vi "Trans_FPGA-old.vi"() -> ()   [LabVIEW 2016]
uses:
  <vilib>/eio/EIONode/EIONode.xnode
  <vilib>/eio/EIOMethodNode/EIOMethodNode.xnode
  <vilib>/LabVIEW Targets/FPGA/cRIO/shared/nicrio_ModuleControls/nicrio_cRIO-9871_BaudRateEnum.ctl
  <vilib>/LabVIEW Targets/FPGA/cRIO/shared/nicrio_ModuleControls/nicrio_cRIO-9871_DataBitsEnum.ctl
  <vilib>/LabVIEW Targets/FPGA/cRIO/shared/nicrio_ModuleControls/nicrio_cRIO-9871_ParityEnum.ctl
  <vilib>/LabVIEW Targets/FPGA/cRIO/shared/nicrio_ModuleControls/nicrio_cRIO-9871_StopBitsEnum.ctl
  <vilib>/eio/EIOPropertyNode/EIOPropertyNode.xnode
  <vilib>/rvi/Analysis/measure/dc-rms/XNode/niFpgaDC-RMS.xnode
  <vilib>/rvi/eio/common/nirviEmuTemplateMethod_errors.vi
  <vilib>/Platform/TimedLoop/XDataNode/wakeup.ctl
  <vilib>/Platform/TimedLoop/XDataNode/XDNodeRunTimeDep.lvlib
  <vilib>/Platform/TimedLoop/XDataNode/nitl_modes.ctl
  <vilib>/Platform/TimedLoop/XDataNode/timing_clust.ctl
  <vilib>/Platform/TimedLoop/XDataNode/XDataNode.xnode
  <vilib>/rvi/FXPMathLib/basic elements/FxpIntAccumulator/XNode/nifxpmath_IntAccumulator.xnode
  <vilib>/rvi/FXPMathLib/FxpMul/XNode/nifxpmath_Multiplier.xnode
  <vilib>/rvi/Analysis/common/codeGenErrors/XNode/niFpgaXNodeCodeGenErrorHandle.vi
  <vilib>/rvi/FXPMathLib/basic elements/FxpIntAccumulator/simVIs/DllFxpIntAccumulator_sub.vi
  <vilib>/rvi/FXPMathLib/basic elements/FxpIntAccumulator/subVIs/nifxpmath_IntAccumulator_SimConfig.ctl
  <vilib>/rvi/FXPMathLib/sim/FxpSim.dll
  <vilib>/rvi/eio/common/nirviEmuTemplatePropertyGet_errors.vi
  <vilib>/rvi/eio/common/nirviEmuTemplatePropertyGet_noerrors.vi
  <vilib>/rvi/eio/common/nirviEmuTemplatePropertySet_errors.vi
  <vilib>/rvi/eio/common/nirviEmuTemplatePropertySet_noerrors.vi
panel:
  in  "analyze ps set array":u8[](array[numeric])=[0, 0, 0, 0, 0, 0, 0, 0, 0, 0]
  out "Data":u8
  out "Timed Out":bool
  out "Analyze read":u8[](array[numeric])
  out "error out":errorcluster
  out "Ion gauge 4":u8[](array[numeric])
  out "Convectron 4":u8[](array[numeric])
  out "Convectron 3":u8[](array[numeric])
  out "Ion gauge 3":u8[](array[numeric])
  out "Ion gauge 2":u8[](array[numeric])
  out "Convectron 2":u8[](array[numeric])
  out "Convectron 1":u8[](array[numeric])
  out "Ion gauge 1":u8[](array[numeric])
  in  "Analog Output":fxp<+/-,26,5>[](array[numeric])=[0.0, 0.0, 0.0, 0.0, 0.0, 0.0, 0.0, 0.0] format="%.23g"
  out "Analog input":fxp<+/-,26,5>[](array[numeric]) format="%.23g"
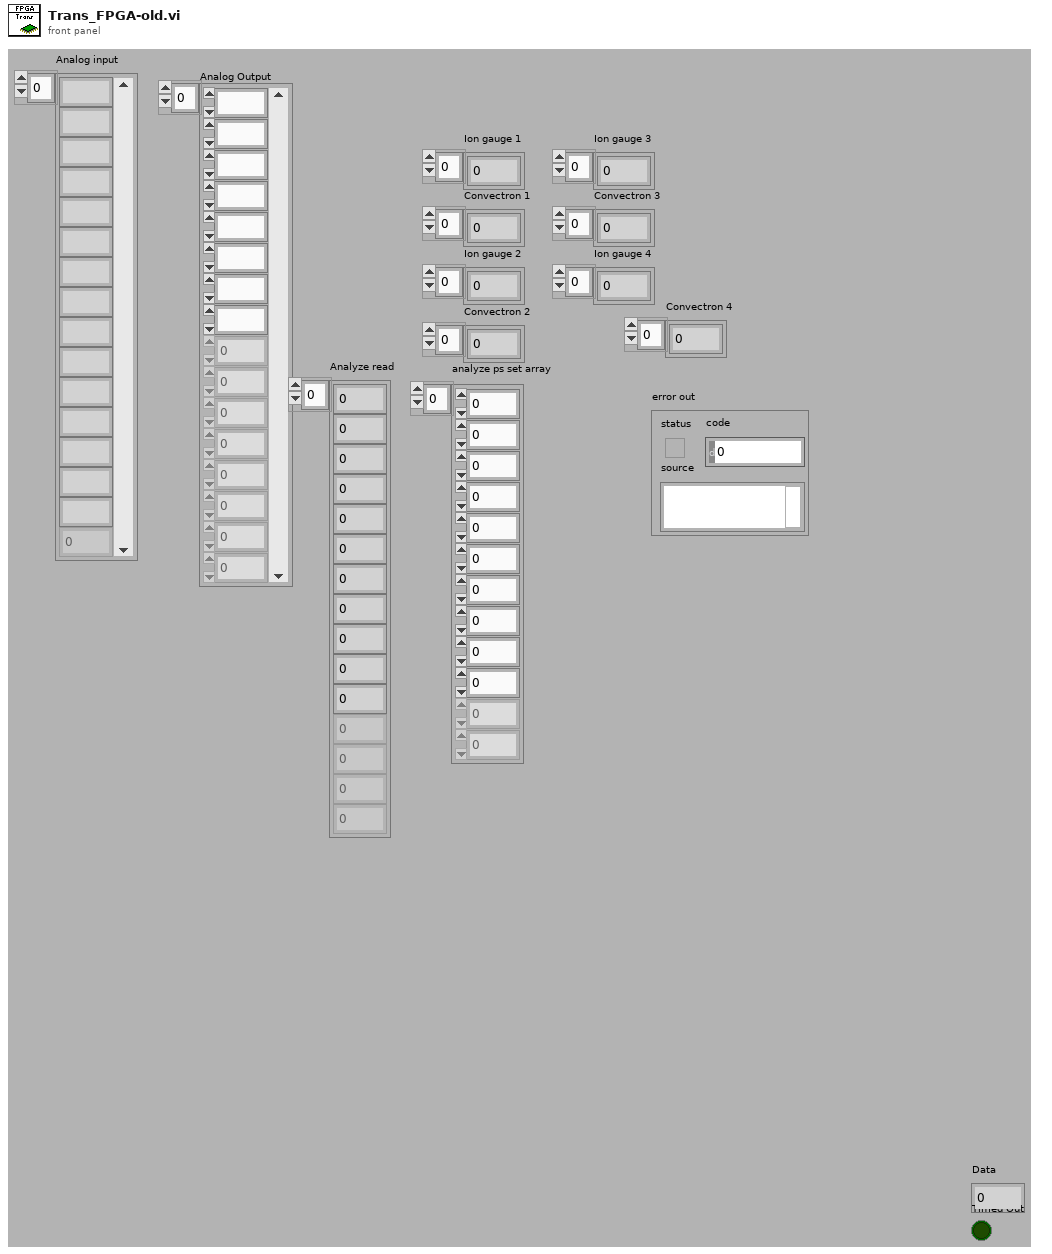
[diagram p1: front panel]
types:
  T1 = typedef "nicrio_cRIO-9871_StopBitsEnum.ctl" = enum8{"1", "1.5", "2"}
  T2 = typedef "nicrio_cRIO-9871_BaudRateEnum.ctl" = enum16{"75 bps", "110 bps", "134 bps", "150 bps", "300 bps", "600 bps", "1200 bps", "1800 bps", "2400 bps", "4800 bps", "7200 bps", "9600 bps", "14.4 kbps", "19.2 kbps", "28.8 kbps", "38.4 kbps", "57.6 kbps", "115.2 kbps", "230.4 kbps", "460.8 kbps", "921.6 kbps"}
  T3 = typedef "nicrio_cRIO-9871_ParityEnum.ctl" = enum8{"None", "Odd", "Even", "Mark", "Space"}
  T4 = typedef "nicrio_cRIO-9871_DataBitsEnum.ctl" = enum8{"5", "6", "7", "8"}
  T5 = typedef "XDNodeRunTimeDep.lvlib/timing_clust.ctl" = cluster{"Expected End [f-1]":u64, "Actual End [f-1]":u64, "Finished Late? [f-1]":bool, "Expected End [i-1]":u64, "Actual End [i-1]":u64, "Finished Late? [i-1]":bool, "Expected Start [i]":u64, "Actual Start [i]":u64, "Expected Start [f]":u64, "Actual Start [f]":u64, "Source Name":string, "Structure Name":string, "Period":i64, "Deadline":i64, "Offset":i64, "Start":i64, "Priority":i32, "Timeout":i32, "Mode":T6, "Wakeup Reason":T7, "Error":errorcluster, "Source Type":string, "Secondary Source Type":string, "Global End Time":u64, "Global Start Time":u64, "Frame Duration":u64, "Iteration Duration":u64, "Assigned CPU":i32, "I/O Scan Engine Mode":u32}
  T6 = typedef "XDNodeRunTimeDep.lvlib/nitl_modes.ctl" = enum32{"No Change", "Process missed periods, maintain original phase", "Discard missed periods, maintain original phase", "Process missed periods, ignore original phase", "Discard missed periods, ignore original phase"}
  T7 = typedef "XDNodeRunTimeDep.lvlib/wakeup.ctl" = enum32{"Normal", "Aborted", "Asynchronous wakeup", "Timing source error", "Timed loop error", "Timeout"}
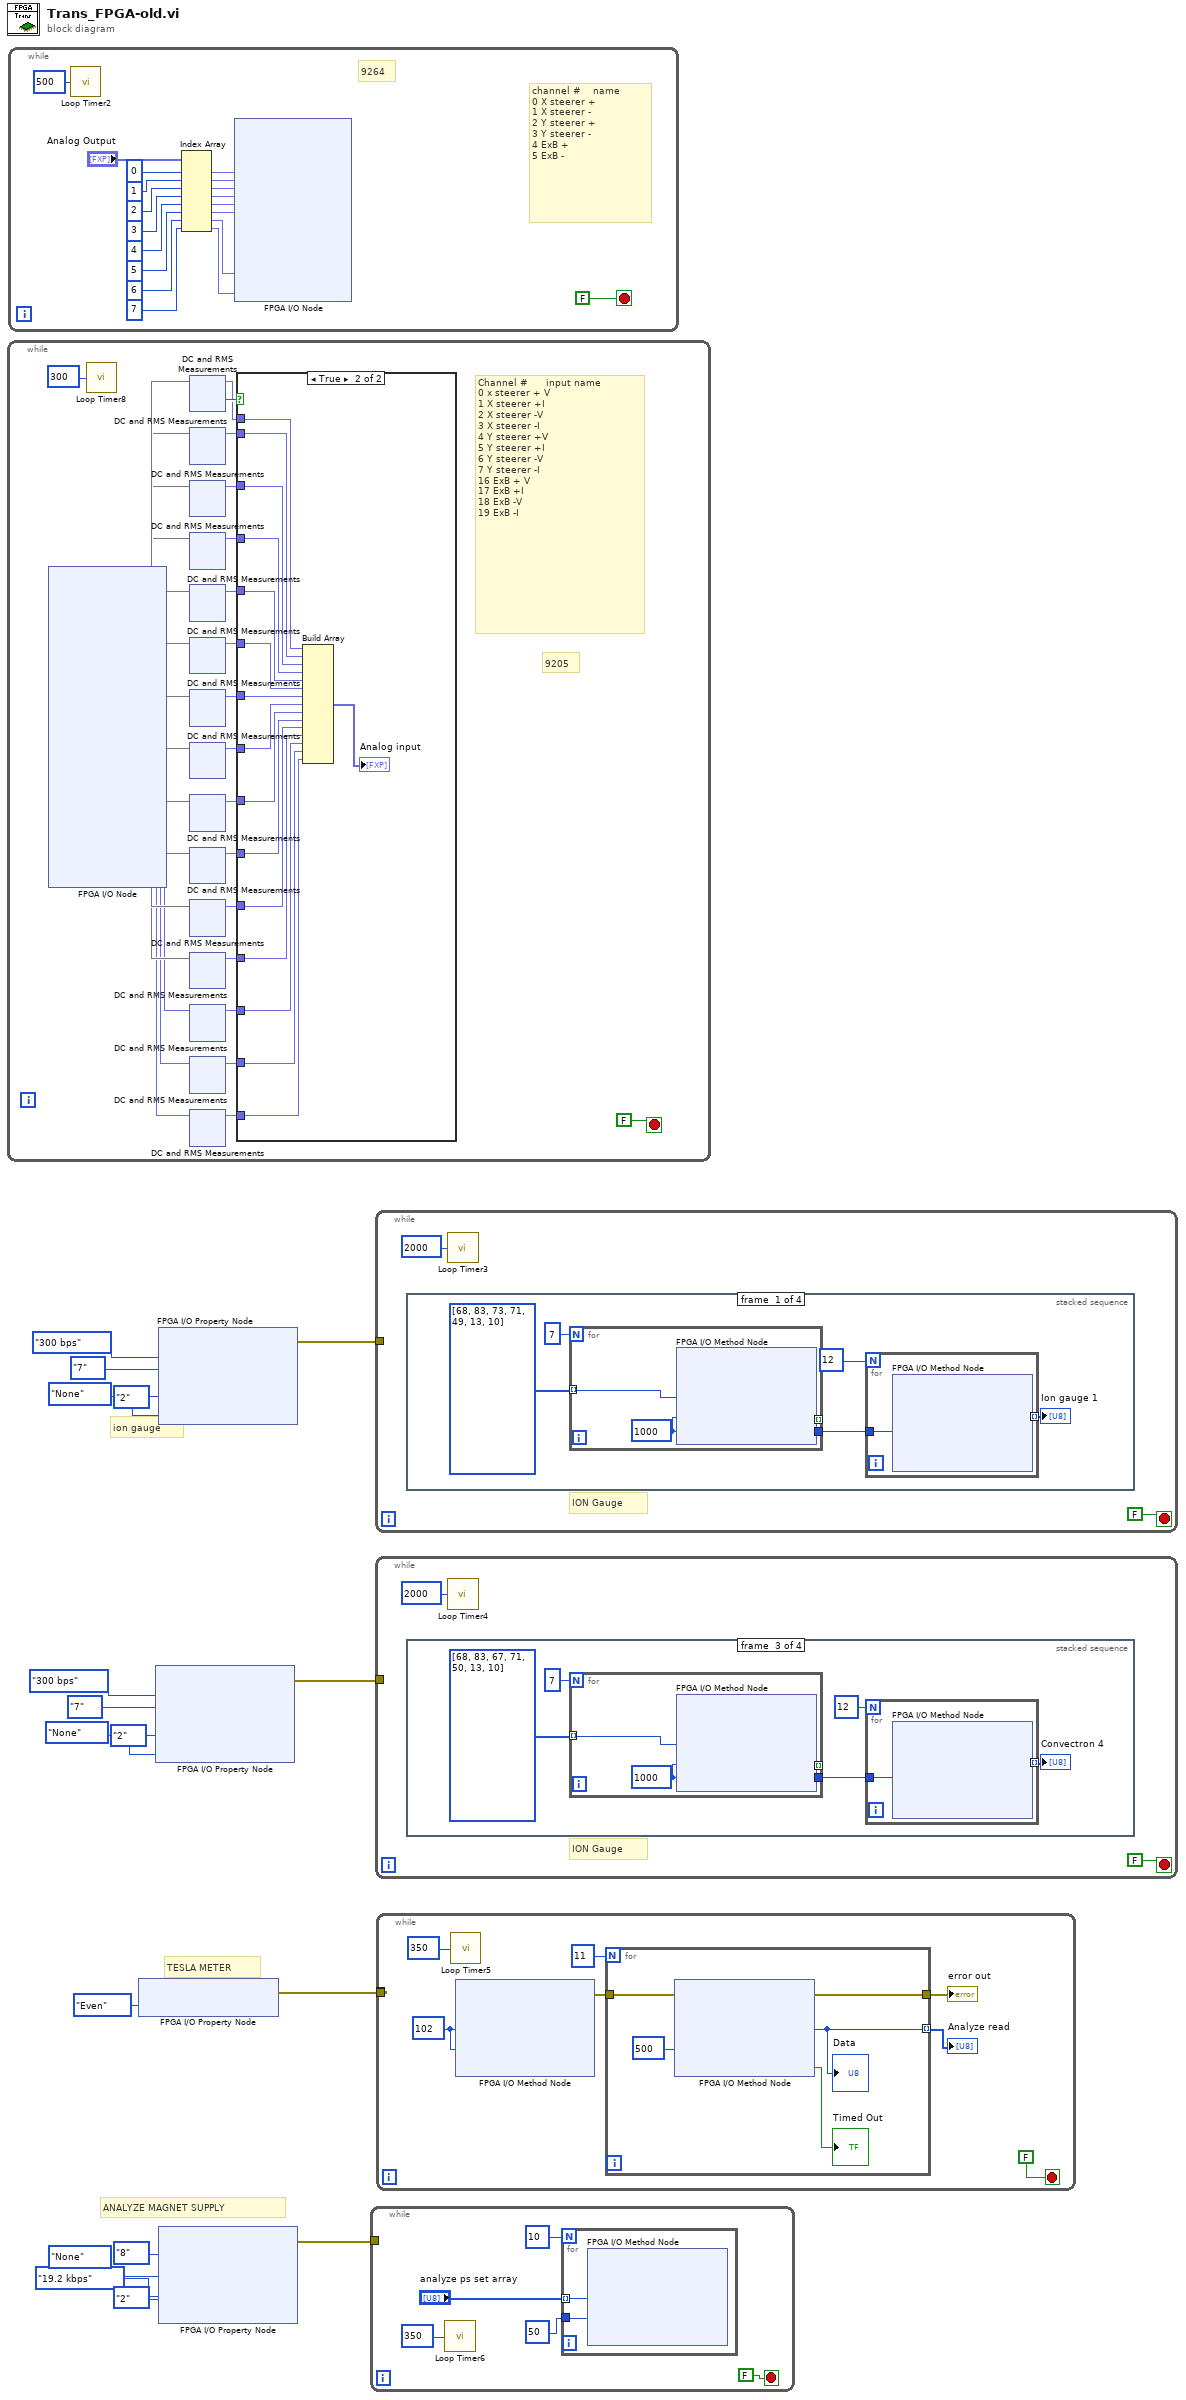
[diagram p0: block diagram]
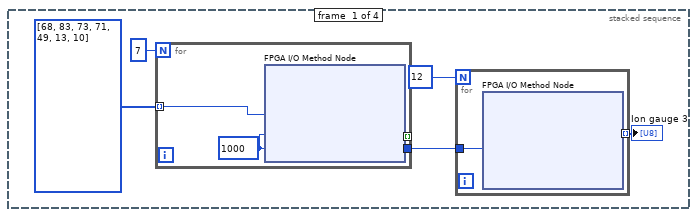
[diagram p3: hidden frame]
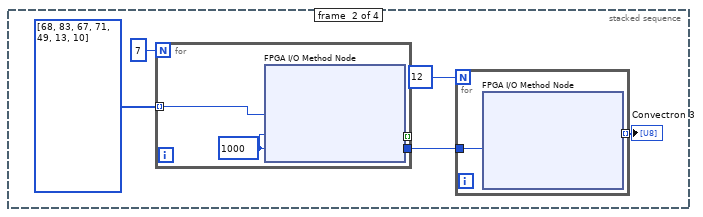
[diagram p4: hidden frame]
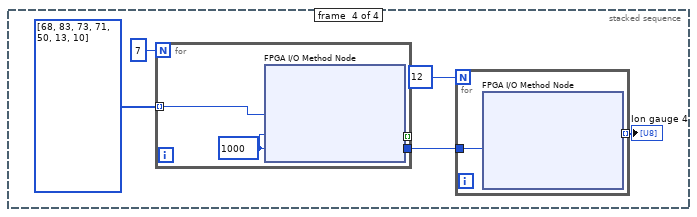
[diagram p5: hidden frame]
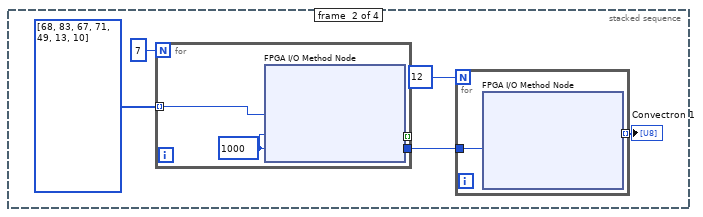
[diagram p6: hidden frame]
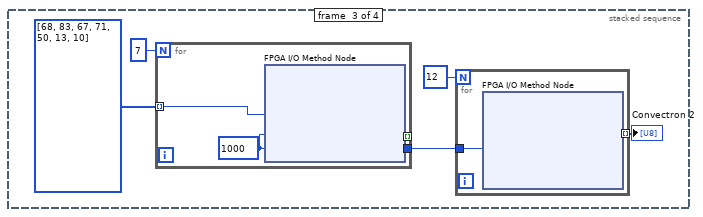
[diagram p7: hidden frame]
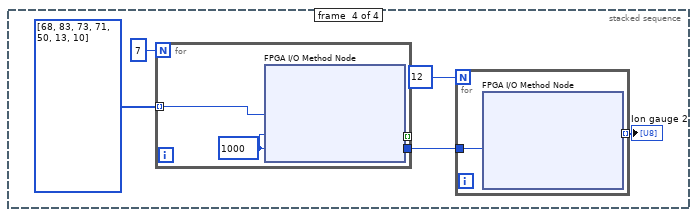
[diagram p8: hidden frame]
diagram:
  # "ANALYZE MAGNET SUPPLY"
  # "TESLA METER"
  # "ion gauge"
  n1 = while {
    stop <- FALSE stop-if-true
    # "Channel #      input name\n0 x steerer + V\n1 X steerer +I\n2 X steerer -V\n3 X steerer -I\n4 Y steerer +V\n5 Y steerer +I\n6 Y steerer -V\n7 Y steerer -I\n16 ExB + V\n17 ExB +I\n18 ExB -V\n19 ExB -I"
    # "9205"
    n2 = xnode "FPGA I/O Node"() -> ("Mod2/AI0"=w47, "Mod2/AI1"=w45, "Mod2/AI2"=w43, "Mod2/AI3"=w41, "Mod2/AI4"=w39, "Mod2/AI5"=w37, "Mod2/AI6"=w35, "Mod2/AI7"=w33, "Mod2/AI16"=w31, "Mod2/AI17"=w29, "Mod2/AI18"=w27, "Mod2/AI19"=w25, "Mod2/AI20"=w23:fxp<+/-,26,5>, "Mod2/AI21"=w21:fxp<+/-,26,5>, "Mod2/AI22"=w19:fxp<+/-,26,5>)  [unwired: 15 in, 15 out]
    n3 = call "Loop Timer8"("Count(Ticks)"=u32 300) -> ()  [unwired: 1 out]
    n4 = xnode "DC and RMS Measurements"("input data"=w47) -> ("DC"=w46:fxp<+/-,26,5>, "output valid"=w48:bool)  [unwired: 1 in]
    n5 = xnode "DC and RMS Measurements"("input data"=w45) -> ("DC"=w44:fxp<+/-,26,5>)  [unwired: 1 in, 1 out]
    n6 = xnode "DC and RMS Measurements"("input data"=w43) -> ("DC"=w42:fxp<+/-,26,5>)  [unwired: 1 in, 1 out]
    n7 = xnode "DC and RMS Measurements"("input data"=w41) -> ("DC"=w40:fxp<+/-,26,5>)  [unwired: 1 in, 1 out]
    n8 = xnode "DC and RMS Measurements"("input data"=w39) -> ("DC"=w38:fxp<+/-,26,5>)  [unwired: 1 in, 1 out]
    n9 = xnode "DC and RMS Measurements"("input data"=w37) -> ("DC"=w36:fxp<+/-,26,5>)  [unwired: 1 in, 1 out]
    n10 = xnode "DC and RMS Measurements"("input data"=w35) -> ("DC"=w34:fxp<+/-,26,5>)  [unwired: 1 in, 1 out]
    n11 = xnode "DC and RMS Measurements"("input data"=w33) -> ("DC"=w32:fxp<+/-,26,5>)  [unwired: 1 in, 1 out]
    n12 = xnode "DC and RMS Measurements"("input data"=w31) -> ("DC"=w30:fxp<+/-,26,5>)  [unwired: 1 in, 1 out]
    n13 = xnode "DC and RMS Measurements"("input data"=w29) -> ("DC"=w28:fxp<+/-,26,5>)  [unwired: 1 in, 1 out]
    n14 = xnode "DC and RMS Measurements"("input data"=w27) -> ("DC"=w26:fxp<+/-,26,5>)  [unwired: 1 in, 1 out]
    n15 = xnode "DC and RMS Measurements"("input data"=w25) -> ("DC"=w24:fxp<+/-,26,5>)  [unwired: 1 in, 1 out]
    n16 = xnode "DC and RMS Measurements"("input data"=w23) -> ("DC"=w22:fxp<+/-,26,5>)  [unwired: 1 in, 1 out]
    n17 = xnode "DC and RMS Measurements"("input data"=w21) -> ("DC"=w20:fxp<+/-,26,5>)  [unwired: 1 in, 1 out]
    n18 = xnode "DC and RMS Measurements"("input data"=w19) -> ("DC"=w18:fxp<+/-,26,5>)  [unwired: 1 in, 1 out]
    n19 = case shown="True" w48 {
      tunnel: w46 -> [_ w226]
      tunnel: w44 -> [_ w225]
      tunnel: w42 -> [_ w224]
      tunnel: w40 -> [_ w223]
      tunnel: w38 -> [_ w222]
      tunnel: w36 -> [_ w221]
      tunnel: w34 -> [_ w220]
      tunnel: w32 -> [_ w219]
      tunnel: w30 -> [_ w218]
      tunnel: w28 -> [_ w217]
      tunnel: w26 -> [_ w216]
      tunnel: w24 -> [_ w215]
      tunnel: w22 -> [_ w214]
      tunnel: w20 -> [_ w213]
      tunnel: w18 -> [_ w212]
      frame False {
      }
      frame True {
        n20 = Build Array(w226, w225, w224, w223, w222, w221, w220, w219, w218, w217, w216, w215, w214, w213, w212) -> (→"Analog input":fxp<+/-,26,5>[])
      }
    }
  }
  n21 = while {
    stop <- FALSE stop-if-true
    # "channel #    name\n0 X steerer +\n1 X steerer -\n2 Y steerer +\n3 Y steerer -\n4 ExB +\n5 ExB -"
    # "9264"
    n22 = call "Loop Timer2"("Count(uSec)"=u32 500 ("Count(Ticks)")) -> ()  [unwired: 1 out]
    n23 = Index Array(array="Analog Output", index #1=0 ("index"), index #2=1 ("index"), index #3=2 ("index"), index #4=3 ("index"), index #5=4 ("index"), index #6=5 ("index"), index #7=6 ("index"), index #8=7 ("index")) -> (element #1=w1278:fxp<+/-,26,5>, element #2=w1277:fxp<+/-,26,5>, element #3=w1276:fxp<+/-,26,5>, element #4=w1275:fxp<+/-,26,5>, element #5=w1270:fxp<+/-,26,5>, element #6=w1269:fxp<+/-,26,5>, element #7=w1268:fxp<+/-,26,5>, element #8=w1267:fxp<+/-,26,5>)
    n24 = xnode "FPGA I/O Node"("Mod1/AO0"=w1278, "Mod1/AO1"=w1277, "Mod1/AO2"=w1276, "Mod1/AO3"=w1275, "Mod1/AO4"=w1270, "Mod1/AO5"=w1269, "Mod1/AO6"=w1268, "Mod1/AO7"=w1267) -> ()  [unwired: 8 in, 8 out]
  }
  n25 = xnode "FPGA I/O Property Node"("Parity"=nicrio_cRIO-9871_ParityEnum."Even") -> ("error out"=w2:errorcluster)  [unwired: 2 in, 1 out]
  n26 = xnode "FPGA I/O Property Node"("Baud Rate"=nicrio_cRIO-9871_BaudRateEnum."300 bps", "Data Bits"=nicrio_cRIO-9871_DataBitsEnum."7", "Parity"=nicrio_cRIO-9871_ParityEnum."None", "Stop Bits"=nicrio_cRIO-9871_StopBitsEnum."2") -> ("error out"=w3:errorcluster)  [unwired: 2 in, 1 out]
  n27 = xnode "FPGA I/O Property Node"("Baud Rate"=nicrio_cRIO-9871_BaudRateEnum."300 bps", "Data Bits"=nicrio_cRIO-9871_DataBitsEnum."7", "Parity"=nicrio_cRIO-9871_ParityEnum."None", "Stop Bits"=nicrio_cRIO-9871_StopBitsEnum."2") -> ("error out"=w4:errorcluster)  [unwired: 2 in, 1 out]
  n28 = xnode "FPGA I/O Property Node"("Data Bits"=nicrio_cRIO-9871_DataBitsEnum."8", "Parity"=nicrio_cRIO-9871_ParityEnum."None", "Baud Rate"=nicrio_cRIO-9871_BaudRateEnum."19.2 kbps", "Stop Bits"=nicrio_cRIO-9871_StopBitsEnum."2") -> ("error out"=w1:errorcluster)  [unwired: 2 in, 1 out]
  n29 = while {
    tunnel: w1 -> [_]
    stop <- FALSE stop-if-true
    n30 = call "Loop Timer6"("Count(mSec)"=u32 350) -> ()  [unwired: 1 out]
    n31 = for {
      N: 10 -> [_]
      tunnel: 50 ("Timeout (ms)") -> [w1292]
      tunnel: "analyze ps set array" -> [w1291] mode=indexing
      n32 = xnode "FPGA I/O Method Node"("Data"=w1291, "Timeout (ms)"=w1292) -> ()  [unwired: 2 in, 3 out]
    }
  }
  n33 = while {
    tunnel: w4 -> [_]
    stop <- FALSE stop-if-true
    # "ION Gauge"
    n34 = stacked-sequence {
      frame #0 {
        n35 = for {
          N: 7 -> [_]
          tunnel: [w1304] -> w1299
          tunnel: [w1303] -> _ mode=indexing
          tunnel: u8[] [68, 83, 73, 71, 49, 13, 10] ("unsigned byte array") -> [w1302] mode=indexing
          w1304 = 1000 ("Timeout (ms)")
          n36 = xnode "FPGA I/O Method Node"("Data"=w1302, "Timeout (ms)"=w1304) -> ("Timed Out"=w1303:bool)  [unwired: 1 in, 1 out]
        }
        n37 = for {
          N: 12 -> [_]
          tunnel: w1299 -> [w1301]
          tunnel: [w1300] -> w1295 mode=indexing
          n38 = xnode "FPGA I/O Method Node"("Timeout (ms)"=w1301) -> ("Data"=w1300:u8)  [unwired: 1 in, 2 out]
        }
        "Ion gauge 1" <- w1295
      }
      frame #1 {
        n39 = for {
          N: 7 -> [_]
          tunnel: [w1314] -> w1309
          tunnel: [w1313] -> _ mode=indexing
          tunnel: u8[] [68, 83, 67, 71, 49, 13, 10] ("unsigned byte array") -> [w1312] mode=indexing
          w1314 = 1000 ("Timeout (ms)")
          n40 = xnode "FPGA I/O Method Node"("Data"=w1312, "Timeout (ms)"=w1314) -> ("Timed Out"=w1313:bool)  [unwired: 1 in, 1 out]
        }
        n41 = for {
          N: 12 -> [_]
          tunnel: w1309 -> [w1311]
          tunnel: [w1310] -> w1305 mode=indexing
          n42 = xnode "FPGA I/O Method Node"("Timeout (ms)"=w1311) -> ("Data"=w1310:u8)  [unwired: 1 in, 2 out]
        }
        "Convectron 1" <- w1305
      }
      frame #2 {
        n43 = for {
          N: 7 -> [_]
          tunnel: [w1324] -> w1319
          tunnel: [w1323] -> _ mode=indexing
          tunnel: u8[] [68, 83, 67, 71, 50, 13, 10] ("unsigned byte array") -> [w1322] mode=indexing
          w1324 = 1000 ("Timeout (ms)")
          n44 = xnode "FPGA I/O Method Node"("Data"=w1322, "Timeout (ms)"=w1324) -> ("Timed Out"=w1323:bool)  [unwired: 1 in, 1 out]
        }
        n45 = for {
          N: 12 -> [_]
          tunnel: w1319 -> [w1321]
          tunnel: [w1320] -> w1315 mode=indexing
          n46 = xnode "FPGA I/O Method Node"("Timeout (ms)"=w1321) -> ("Data"=w1320:u8)  [unwired: 1 in, 2 out]
        }
        "Convectron 2" <- w1315
      }
      frame #3 {
        n47 = for {
          N: 7 -> [_]
          tunnel: [w1334] -> w1329
          tunnel: [w1333] -> _ mode=indexing
          tunnel: u8[] [68, 83, 73, 71, 50, 13, 10] ("unsigned byte array") -> [w1332] mode=indexing
          w1334 = 1000 ("Timeout (ms)")
          n48 = xnode "FPGA I/O Method Node"("Data"=w1332, "Timeout (ms)"=w1334) -> ("Timed Out"=w1333:bool)  [unwired: 1 in, 1 out]
        }
        n49 = for {
          N: 12 -> [_]
          tunnel: w1329 -> [w1331]
          tunnel: [w1330] -> w1325 mode=indexing
          n50 = xnode "FPGA I/O Method Node"("Timeout (ms)"=w1331) -> ("Data"=w1330:u8)  [unwired: 1 in, 2 out]
        }
        "Ion gauge 2" <- w1325
      }
    }
    n51 = call "Loop Timer3"("Count(mSec)"=u32 2000 ("Count(Ticks)")) -> ()  [unwired: 1 out]
  }
  n52 = while {
    tunnel: w3 -> [_]
    stop <- FALSE stop-if-true
    # "ION Gauge"
    n53 = stacked-sequence {
      frame #0 {
        n54 = for {
          N: 7 -> [_]
          tunnel: [w1346] -> w1341
          tunnel: [w1345] -> _ mode=indexing
          tunnel: u8[] [68, 83, 73, 71, 49, 13, 10] ("unsigned byte array") -> [w1344] mode=indexing
          w1346 = 1000 ("Timeout (ms)")
          n55 = xnode "FPGA I/O Method Node"("Data"=w1344, "Timeout (ms)"=w1346) -> ("Timed Out"=w1345:bool)  [unwired: 1 in, 1 out]
        }
        n56 = for {
          N: 12 -> [_]
          tunnel: w1341 -> [w1343]
          tunnel: [w1342] -> w1337 mode=indexing
          n57 = xnode "FPGA I/O Method Node"("Timeout (ms)"=w1343) -> ("Data"=w1342:u8)  [unwired: 1 in, 2 out]
        }
        "Ion gauge 3" <- w1337
      }
      frame #1 {
        n58 = for {
          N: 7 -> [_]
          tunnel: [w1356] -> w1351
          tunnel: [w1355] -> _ mode=indexing
          tunnel: u8[] [68, 83, 67, 71, 49, 13, 10] ("unsigned byte array") -> [w1354] mode=indexing
          w1356 = 1000 ("Timeout (ms)")
          n59 = xnode "FPGA I/O Method Node"("Data"=w1354, "Timeout (ms)"=w1356) -> ("Timed Out"=w1355:bool)  [unwired: 1 in, 1 out]
        }
        n60 = for {
          N: 12 -> [_]
          tunnel: w1351 -> [w1353]
          tunnel: [w1352] -> w1347 mode=indexing
          n61 = xnode "FPGA I/O Method Node"("Timeout (ms)"=w1353) -> ("Data"=w1352:u8)  [unwired: 1 in, 2 out]
        }
        "Convectron 3" <- w1347
      }
      frame #2 {
        n62 = for {
          N: 7 -> [_]
          tunnel: [w1366] -> w1361
          tunnel: [w1365] -> _ mode=indexing
          tunnel: u8[] [68, 83, 67, 71, 50, 13, 10] ("unsigned byte array") -> [w1364] mode=indexing
          w1366 = 1000 ("Timeout (ms)")
          n63 = xnode "FPGA I/O Method Node"("Data"=w1364, "Timeout (ms)"=w1366) -> ("Timed Out"=w1365:bool)  [unwired: 1 in, 1 out]
        }
        n64 = for {
          N: 12 -> [_]
          tunnel: w1361 -> [w1363]
          tunnel: [w1362] -> w1357 mode=indexing
          n65 = xnode "FPGA I/O Method Node"("Timeout (ms)"=w1363) -> ("Data"=w1362:u8)  [unwired: 1 in, 2 out]
        }
        "Convectron 4" <- w1357
      }
      frame #3 {
        n66 = for {
          N: 7 -> [_]
          tunnel: [w1376] -> w1371
          tunnel: [w1375] -> _ mode=indexing
          tunnel: u8[] [68, 83, 73, 71, 50, 13, 10] ("unsigned byte array") -> [w1374] mode=indexing
          w1376 = 1000 ("Timeout (ms)")
          n67 = xnode "FPGA I/O Method Node"("Data"=w1374, "Timeout (ms)"=w1376) -> ("Timed Out"=w1375:bool)  [unwired: 1 in, 1 out]
        }
        n68 = for {
          N: 12 -> [_]
          tunnel: w1371 -> [w1373]
          tunnel: [w1372] -> w1367 mode=indexing
          n69 = xnode "FPGA I/O Method Node"("Timeout (ms)"=w1373) -> ("Data"=w1372:u8)  [unwired: 1 in, 2 out]
        }
        "Ion gauge 4" <- w1367
      }
    }
    n70 = call "Loop Timer4"("Count(mSec)"=u32 2000 ("Count(Ticks)")) -> ()  [unwired: 1 out]
  }
  n71 = while {
    tunnel: [w1377] -> _
    tunnel: w2 -> [w1377]
    stop <- FALSE stop-if-true
    w1381 = u8 102 ("Data")
    n72 = call "Loop Timer5"("Count(mSec)"=u32 350) -> ()  [unwired: 1 out]
    n73 = xnode "FPGA I/O Method Node"("Data"=w1381, "Timeout (ms)"=w1381) -> ("error out"=w1380:errorcluster)  [unwired: 2 in, 2 out]
    n74 = for {
      N: 11 ("Numeric 3") -> [_]
      tunnel: [w1387] -> w1382 mode=indexing
      tunnel: w1380 -> [w1386]
      tunnel: [w1385] -> w1379
      n75 = xnode "FPGA I/O Method Node"("error in"=w1386, "Timeout (ms)"=500) -> ("error out"=w1385:errorcluster, "Data"=w1387:u8, "Timed Out"=→"Timed Out":bool)  [unwired: 1 in, 1 out]
      "Data" <- w1387
    }
    "Analyze read" <- w1382
    "error out" <- w1379
  }
